vi "export_DFX.vi"(10 "Q1":sgl, 11 "vacuum":sgl) -> ()   [LabVIEW 2012]
uses:
  FT_HMI.llb/GLOBAL_GEN.vi
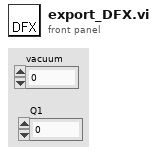
[diagram p1: front panel]
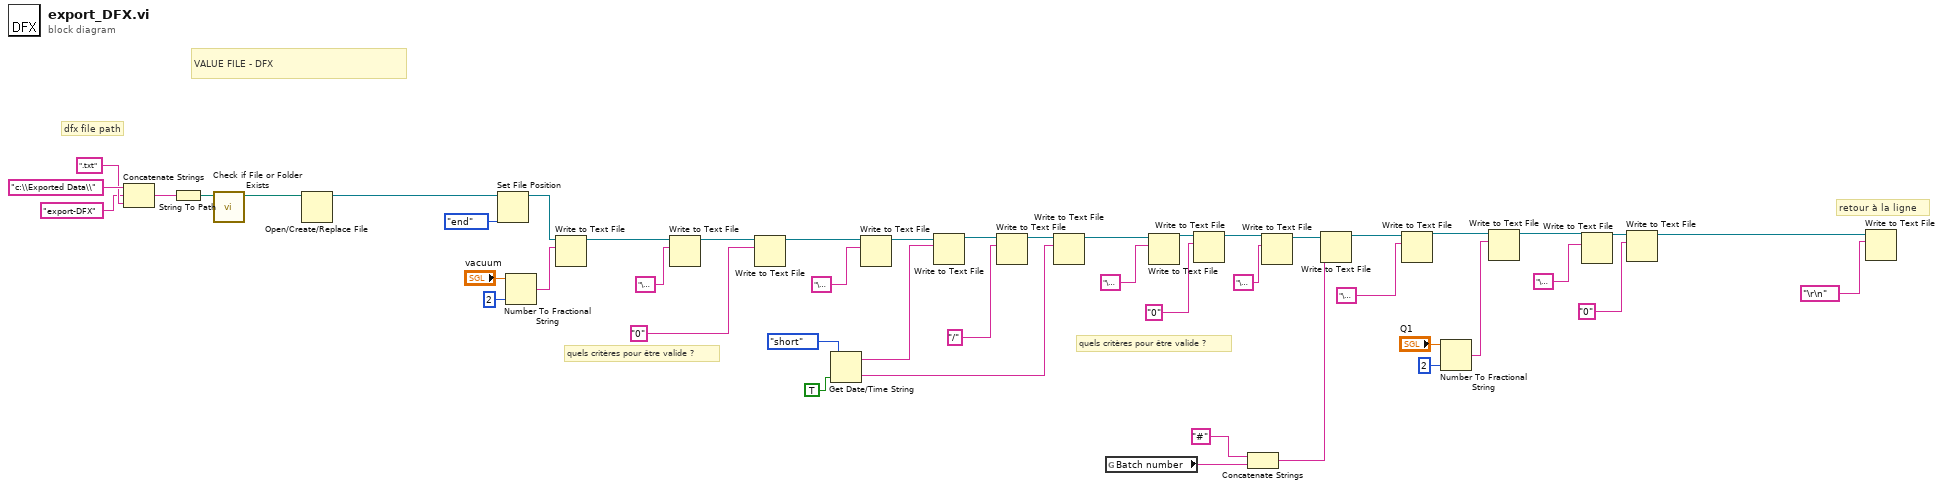
[diagram p0: block diagram]
diagram:
  # "quels critères pour être valide ?"
  # "dfx file path"
  # "VALUE FILE - DFX"
  # "quels critères pour être valide ?"
  # "retour à la ligne"
  n1 = Concatenate Strings("c:\\Exported Data\\", "export-DFX" ("string"), ".txt") -> (w45:string)
  n2 = String To Path(string=w45) -> (path=w47:path)
  n3 = call <vilib>:"Check if File or Folder Exists.vi"("path"=w47) -> ("dup path"=w19:path)  [unwired: 8 in, 2 out]
  n4 = Open/Create/Replace File(file path (use dialog)=w19) -> (refnum out=w17:refnum<file>)  [unwired: 5 in, 2 out]
  n5 = Set File Position(refnum=w17, from (0:start)=enum16{"start", "end", "current"}."end") -> (refnum out=w16:refnum<file>)  [unwired: 2 in, 1 out]
  n6 = Number To Fractional String(number="vacuum", precision (6)=i16 2 ("width (-)")) -> (F-format string=w20:string)  [unwired: 2 in]
  n7 = Write to Text File(file (use dialog)=w16, text=w20) -> (refnum out=w43:refnum<file>)  [unwired: 2 in, 2 out]
  n8 = Write to Text File(file (use dialog)=w43, text="\u0014") -> (refnum out=w40:refnum<file>)  [unwired: 2 in, 2 out]
  n9 = Write to Text File(file (use dialog)=w40, text="0") -> (refnum out=w39:refnum<file>)  [unwired: 2 in, 2 out]
  n10 = Get Date/Time String(date format (0)=enum16{"short", "long", "abbreviated"}."short", want seconds? (F)=TRUE) -> (date string=w35:string, time string=w34:string)  [unwired: 1 in]
  n11 = Write to Text File(file (use dialog)=w39, text="\u0014") -> (refnum out=w36:refnum<file>)  [unwired: 2 in, 2 out]
  n12 = Write to Text File(file (use dialog)=w36, text=w35) -> (refnum out=w31:refnum<file>)  [unwired: 2 in, 2 out]
  n13 = Write to Text File(file (use dialog)=w31, text="/") -> (refnum out=w30:refnum<file>)  [unwired: 2 in, 2 out]
  n14 = Write to Text File(file (use dialog)=w30, text=w34) -> (refnum out=w33:refnum<file>)  [unwired: 2 in, 2 out]
  n15 = global read "GLOBAL_GEN.vi" "Batch number"() -> (w26:string)
  n16 = Write to Text File(file (use dialog)=w33, text="\u0014") -> (refnum out=w27:refnum<file>)  [unwired: 2 in, 2 out]
  n17 = Write to Text File(file (use dialog)=w27, text="0") -> (refnum out=w11:refnum<file>)  [unwired: 2 in, 2 out]
  n18 = Concatenate Strings("#" ("string"), w26) -> (w24:string)
  n19 = Write to Text File(file (use dialog)=w11, text="\u0014") -> (refnum out=w10:refnum<file>)  [unwired: 2 in, 2 out]
  n20 = Write to Text File(file (use dialog)=w10, text=w24) -> (refnum out=w23:refnum<file>)  [unwired: 2 in, 2 out]
  n21 = Write to Text File(file (use dialog)=w23, text="\u000f") -> (refnum out=w6:refnum<file>)  [unwired: 2 in, 2 out]
  n22 = Number To Fractional String(number="Q1", precision (6)=i16 2 ("width (-)")) -> (F-format string=w9:string)  [unwired: 2 in]
  n23 = Write to Text File(file (use dialog)=w6, text=w9) -> (refnum out=w2:refnum<file>)  [unwired: 2 in, 2 out]
  n24 = Write to Text File(file (use dialog)=w2, text="\u0014") -> (refnum out=w3:refnum<file>)  [unwired: 2 in, 2 out]
  n25 = Write to Text File(file (use dialog)=w3, text="0") -> (refnum out=w1:refnum<file>)  [unwired: 2 in, 2 out]
  n26 = Write to Text File(file (use dialog)=w1, text="\r\n") -> ()  [unwired: 2 in, 3 out]
